vi "Sorted Archived Data.vi"(0 "Dataset Source":T1, 5 "Transactions":string[](array[string])) -> (4 "LBCB 1":dbl[](array[numeric]), 6 "LBCB 2":dbl[](array[numeric]), 8 "External":dbl[](array[numeric]), 10 "Combined":dbl[](array[numeric]))   [LabVIEW 2013]
uses:
  Global Data/Dataset Source.ctl
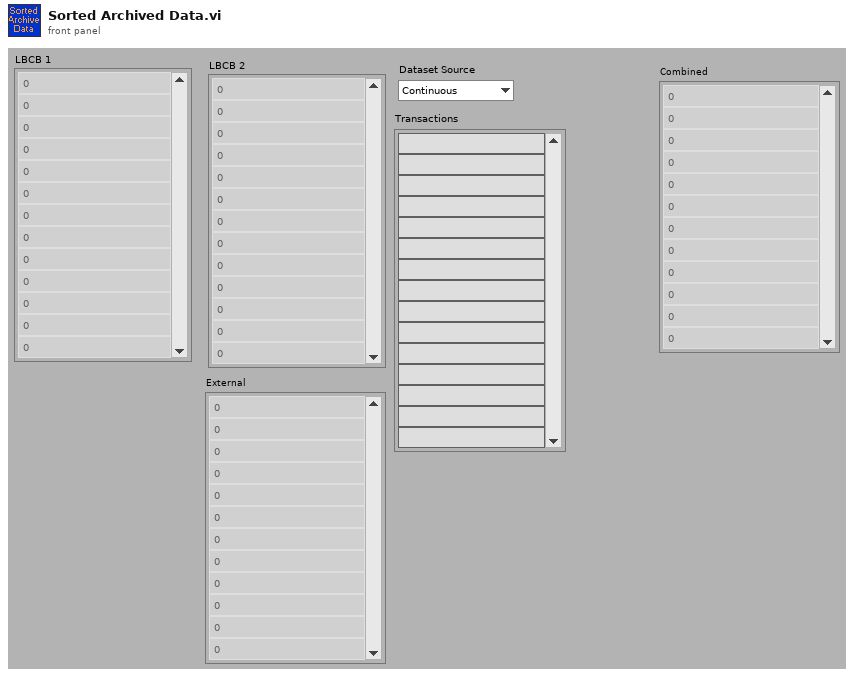
[diagram p1: front panel]
types:
  T1 = typedef "Dataset Source.ctl" = enum16{"Continuous", "Hold", "ED", "Volts", "Offsets", "Increments"}
  T2 = typedef "Source Group Type.ctl" = enum16{"LBCB1", "LBCB2", "Consolidated", "External"}
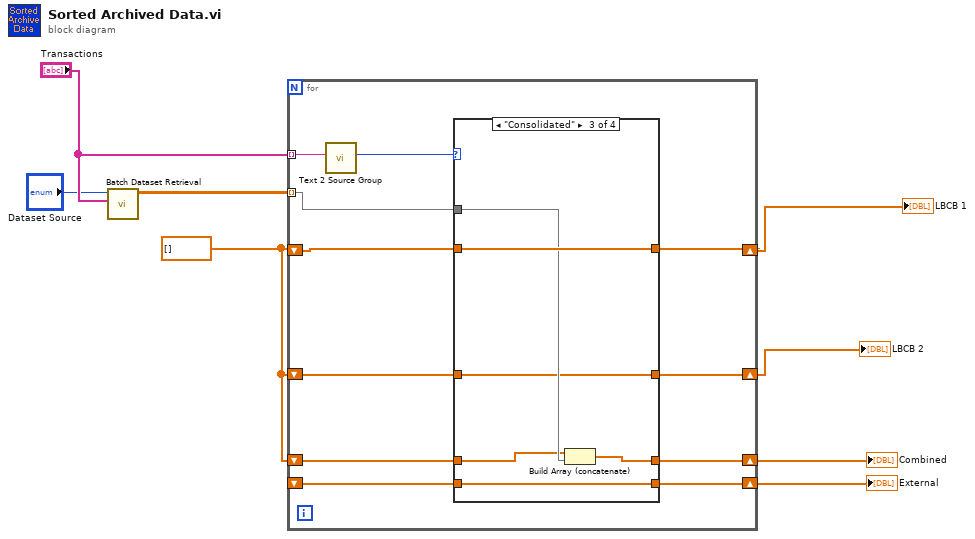
[diagram p0: block diagram]
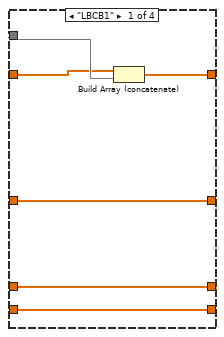
[diagram p2: hidden frame]
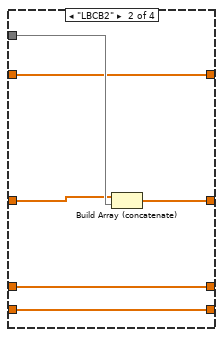
[diagram p3: hidden frame]
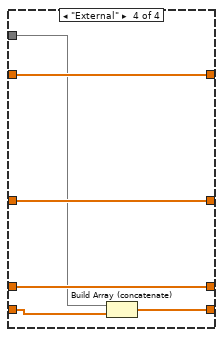
[diagram p4: hidden frame]
diagram:
  w5 = dbl[] []
  n1 = call "Batch Dataset Retrieval.vi"("Dataset Source"="Dataset Source", "Transactions"="Transactions") -> ("Data"=w8:dbl[][])  [unwired: 7 in, 1 out]
  n2 = for {
    tunnel: w8 -> [w19] mode=indexing
    tunnel: "Transactions" -> [w12] mode=indexing
    shift-right: [w18] -> w7
    shift-left: w5 -> [w17]
    shift-right: [w16] -> w4
    shift-left: w5 -> [w15]
    shift-right: [w14] -> w6
    shift-left: w5 -> [w13]
    shift-right: [w9] -> w1
    shift-left: _ -> [w10]
    n3 = call "Text 2 Source Group.vi"("Text"=w12) -> ("Source Group"=w11:T2)  [unwired: 10 in]
    n4 = case shown="\"Consolidated\"" w11 {
      tunnel: w19 -> [w25 w31 w36 w40]
      tunnel: [w24 w28 w37 w43] -> w18
      tunnel: w17 -> [w23 w28 w37 w43]
      tunnel: [w22 w30 w33 w41] -> w16
      tunnel: w15 -> [w22 w29 w33 w41]
      tunnel: [w21 w27 w35 w42] -> w14
      tunnel: w13 -> [w21 w27 w34 w42]
      tunnel: [w20 w26 w32 w39] -> w9
      tunnel: w10 -> [w20 w26 w32 w38]
      frame "LBCB1" {
        n5 = Build Array (concatenate)(w23, w25) -> (w24:dbl[])
      }
      frame "LBCB2" {
        n6 = Build Array (concatenate)(w29, w31) -> (w30:dbl[])
      }
      frame "Consolidated" {
        n7 = Build Array (concatenate)(w34, w36) -> (w35:dbl[])
      }
      frame "External" {
        n8 = Build Array (concatenate)(w40, w38) -> (w39:dbl[])
      }
    }
  }
  "Combined" <- w6
  "LBCB 1" <- w7
  "LBCB 2" <- w4
  "External" <- w1
